vi "Projectile Motion 3.vi"() -> ()   [LabVIEW 2016]
panel:
  out "XY Graph":cluster{dbl[], dbl[]}(graph)
  in  "Boolean":bool
  in  "Number of Points":i32=5
  in  "Y Velocity Array":dbl[](array[numeric])
  in  "X Velocity Array":dbl[](array[numeric])
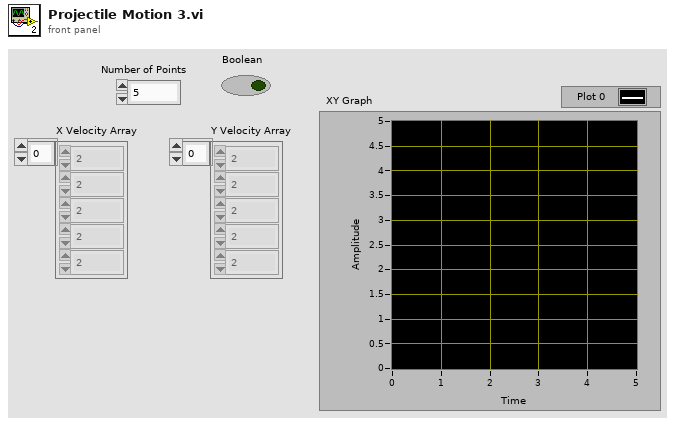
[diagram p1: front panel]
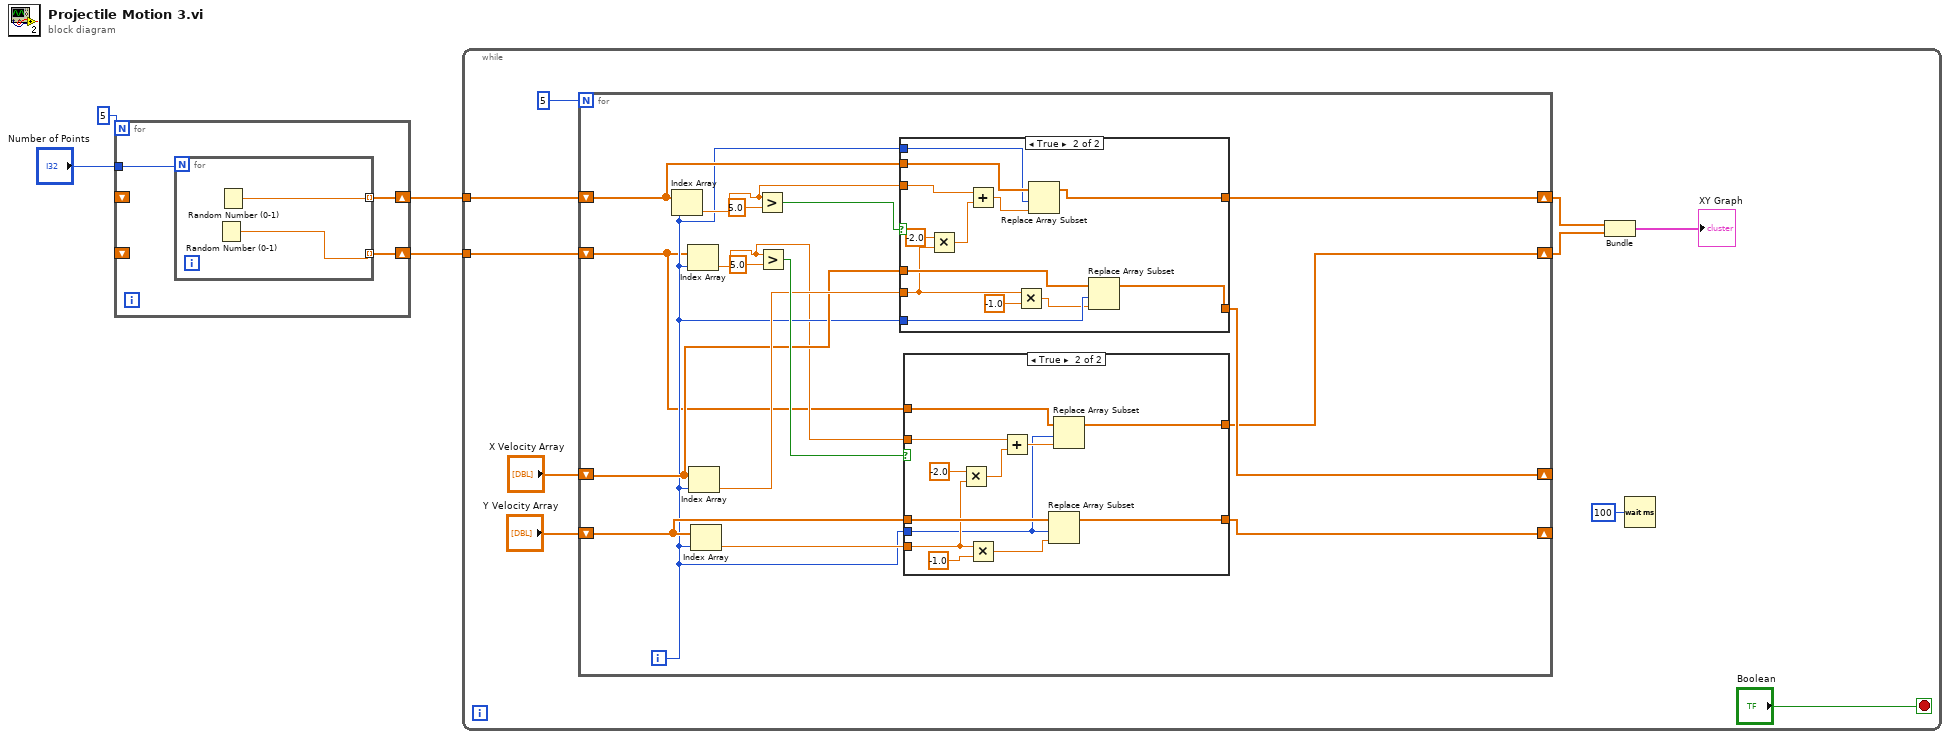
[diagram p0: block diagram]
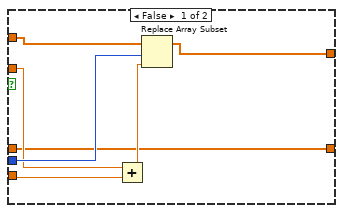
[diagram p2: hidden frame]
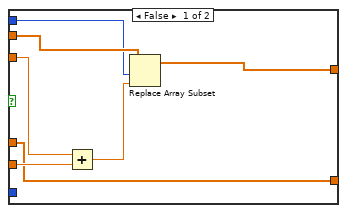
[diagram p3: hidden frame]
diagram:
  n1 = for {
    N: 5 -> [_]
    shift-right: [w7] -> w2
    shift-left: _ -> [_]
    shift-right: [w6] -> w3
    shift-left: _ -> [_]
    tunnel: "Number of Points" -> [w5]
    n2 = for {
      N: w5 -> [_]
      tunnel: [w9] -> w7 mode=indexing
      tunnel: [w8] -> w6 mode=indexing
      n3 = Random Number (0-1)() -> (number: 0 to 1=w8:dbl)
      n4 = Random Number (0-1)() -> (number: 0 to 1=w9:dbl)
    }
  }
  n5 = while {
    tunnel: w3 -> [w19]
    tunnel: w2 -> [w18]
    stop <- "Boolean" stop-if-true
    n6 = for {
      N: 5 -> [_]
      shift-right: [w28] -> _
      shift-left: "X Velocity Array" -> [w29]
      shift-right: [w24] -> _
      shift-left: "Y Velocity Array" -> [w26]
      shift-right: [w21] -> w16
      shift-left: w18 -> [w31]
      shift-right: [w20] -> w15
      shift-left: w19 -> [w22]
      i -> [w25]
      n7 = Index Array(array=w31, index=w25) -> (element=w30:dbl)
      n8 = Index Array(array=w22, index=w25) -> (element=w23:dbl)
      n9 = Index Array(array=w29, index=w25) -> (element=w32:dbl)
      n10 = Index Array(array=w26, index=w25) -> (element=w27:dbl)
      n11 = Greater?(x=w30, y=5.0) -> (0:w34:bool)
      n12 = Greater?(x=w23, y=5.0) -> (0:w33:bool)
      n13 = case shown="True" w34 {
        tunnel: w32 -> [w59 w69]
        tunnel: w31 -> [w62 w66]
        tunnel: w25 -> [w61 w64]
        tunnel: w30 -> [w60 w70]
        tunnel: [w57 w63] -> w21
        tunnel: w29 -> [w56 w74]
        tunnel: w25 -> [_ w73]
        tunnel: [w56 w71] -> w28
        frame False {
          n14 = Add(x=w60, y=w59) -> (x+y=w58:dbl)
          n15 = Replace Array Subset(array=w62, new element=w58, index=w61) -> (w57:dbl[])
        }
        frame True {
          n16 = Multiply(x=-2.0, y=w69) -> (x*y=w67:dbl)
          n17 = Add(x=w70, y=w67) -> (x+y=w65:dbl)
          n18 = Multiply(x=w69, y=-1.0) -> (x*y=w72:dbl)
          n19 = Replace Array Subset(array=w66, new element=w65, index=w64) -> (w63:dbl[])
          n20 = Replace Array Subset(array=w74, new element=w72, index=w73) -> (w71:dbl[])
        }
      }
      n21 = case shown="True" w33 {
        tunnel: w27 -> [w41 w50]
        tunnel: w26 -> [w37 w54]
        tunnel: w25 -> [w42 w46]
        tunnel: [w37 w52] -> w24
        tunnel: w23 -> [w38 w48]
        tunnel: w22 -> [w43 w45]
        tunnel: [w39 w44] -> w20
        frame False {
          n22 = Add(x=w38, y=w41) -> (x+y=w40:dbl)
          n23 = Replace Array Subset(array=w43, new element=w40, index=w42) -> (w39:dbl[])
        }
        frame True {
          n24 = Multiply(x=-2.0, y=w50) -> (x*y=w49:dbl)
          n25 = Multiply(x=w50, y=-1.0) -> (x*y=w53:dbl)
          n26 = Add(x=w48, y=w49) -> (x+y=w47:dbl)
          n27 = Replace Array Subset(array=w54, new element=w53, index=w46) -> (w52:dbl[])
          n28 = Replace Array Subset(array=w45, new element=w47, index=w46) -> (w44:dbl[])
        }
      }
    }
    n29 = Bundle(w16, w15) -> (→"XY Graph":cluster{dbl[], dbl[]})  [unwired: 1 in]
    n30 = Wait (ms)(milliseconds to wait=u32 100) -> ()  [unwired: 1 out]
  }
